vi "Encoder read task.vi"() -> (0 "error out":errorcluster, 3 "task out":refnum<k21>)   [LabVIEW 2017]
uses:
  <vilib>/DAQmx/create/channels.llb/DAQmx Create Channel (CI-Position-Angular Encoder).vi
  <resource>/objmgr/daqmx.rc
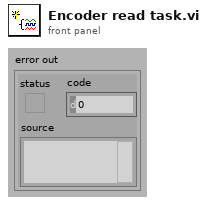
[diagram p1: front panel]
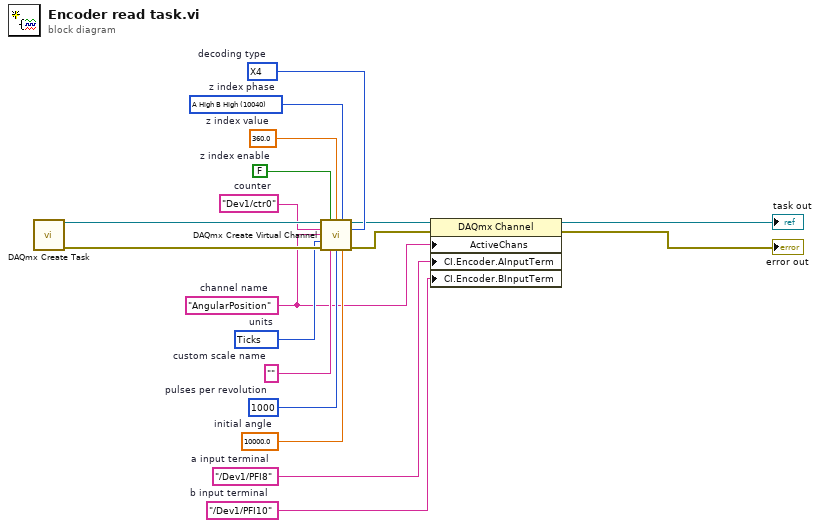
[diagram p0: block diagram]
diagram:
  w3 = "/Dev1/PFI10"  # b input terminal
  w4 = "/Dev1/PFI8"  # a input terminal
  w12 = 10304 items=["Degrees"=10146, "Radians"=10273, "Ticks"=10304, "From Custom Scale"=10065]  # units
  w8 = 10092 items=["X1"=10090, "X2"=10091, "X4"=10092, "Two Pulse Counting"=10313]  # decoding type
  w9 = 10000.0  # initial angle
  w10 = u32 1000  # pulses per revolution
  w11 = ""  # custom scale name
  w13 = 10040 items=["A High B High"=10040, "A High B Low"=10041, "A Low B High"=10042, "A Low B Low"=10043]  # z index phase
  w14 = 360.0  # z index value
  w6 = FALSE  # z index enable
  w5 = "AngularPosition"  # channel name
  w16 = "Dev1/ctr0"  # counter
  n1 = call <vilib>:"DAQmx Create Task.vi"() -> ("task out"=w17:refnum<k21>, "error out"=w18:errorcluster)  [unwired: 14 in]
  n2 = call-poly <vilib>:"DAQmx Create Virtual Channel.vi"("task in"=w17, "z index enable"=w6, "z index value"=w14, "z index phase"=w13, "counter"=w16, "decoding type"=w8, "name to assign"=w5, "units"=w12, "error in"=w18, "custom scale name"=w11, "pulses per revolution"=w10, "initial angle"=w9) -> ("task out"=w7:refnum<k21>, "error out"=w15:errorcluster)  [unwired: 2 in]
  n3 = property class="DAQmx Channel"(reference=w7, error in=w15, "ActiveChans"=w5, "CI.Encoder.AInputTerm"=w4, "CI.Encoder.BInputTerm"=w3) -> (reference out=→"task out":refnum<k21>, error out=→"error out":errorcluster)
